vi "Rotate.vi"(2 "背景":dbl[][](array[numeric]), 3 "point":cluster{"x":i16, "y":i16} caption="位置", 4 "宽度":dbl, 5 "输入":cluster{"编号":i8, "方块":i32[][]}) -> (0 "输出":cluster{"编号":i8, "方块":i32[][]}, 1 "point 2":cluster{"x":i16, "y":i16} caption="新位置")   [LabVIEW 2010]
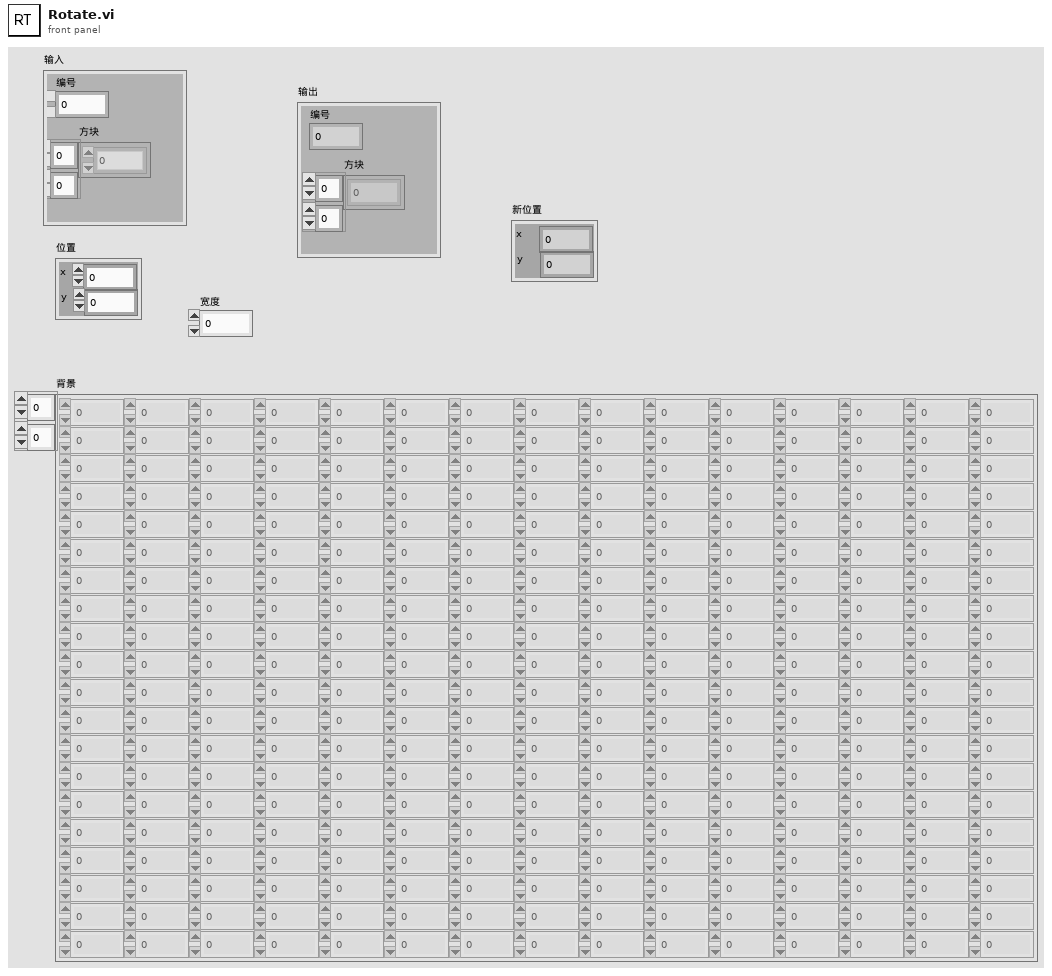
[diagram p1: front panel]
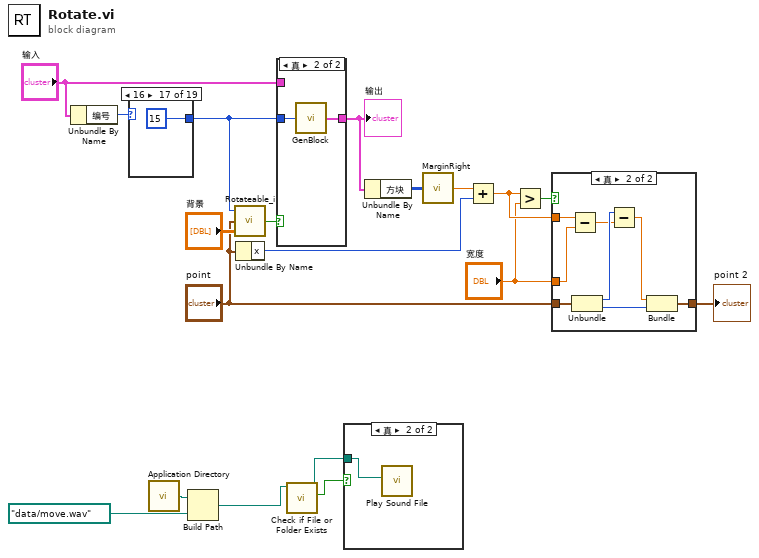
[diagram p0: block diagram]
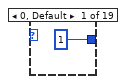
[diagram p5: hidden frame]
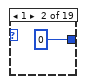
[diagram p6: hidden frame]
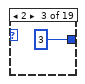
[diagram p7: hidden frame]
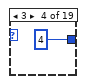
[diagram p8: hidden frame]
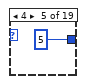
[diagram p9: hidden frame]
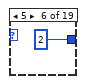
[diagram p10: hidden frame]
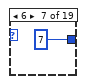
[diagram p11: hidden frame]
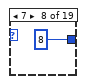
[diagram p12: hidden frame]
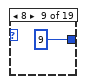
[diagram p13: hidden frame]
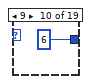
[diagram p14: hidden frame]
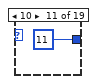
[diagram p15: hidden frame]
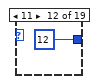
[diagram p16: hidden frame]
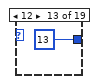
[diagram p17: hidden frame]
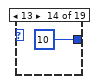
[diagram p18: hidden frame]
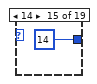
[diagram p19: hidden frame]
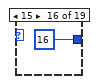
[diagram p20: hidden frame]
diagram:
  n1 = Unbundle By Name("输入") -> ("编号"=w16:i8)
  n2 = case shown="16" w16 {
    tunnel: [1 0 3 4 5 2 7 8 9 6 11 12 13 10 14 16 15 18 17] -> w15
    frame 0, Default {
    }
    frame 1 {
    }
    frame 2 {
    }
    frame 3 {
    }
    frame 4 {
    }
    frame 5 {
    }
    frame 6 {
    }
    frame 7 {
    }
    frame 8 {
    }
    frame 9 {
    }
    frame 10 {
    }
    frame 11 {
    }
    frame 12 {
    }
    frame 13 {
    }
    frame 14 {
    }
    frame 15 {
    }
    frame 16 {
    }
    frame 17 {
    }
    frame 18 {
    }
  }
  n3 = call <vilib>:"Application Directory.vi"() -> ("Application Directory"=w4:path)
  n4 = Build Path(base path=w4, name or relative path=path "data/move.wav") -> (appended path=w3:path)
  n5 = call "Rotateable_i.vi"("背景"="背景", "point"="point", "编号"=w15) -> ("Rotateable"=w18:bool)
  n6 = Unbundle By Name("point") -> ("x"=w12:i16)
  n7 = case shown="真" w18 {
    tunnel: [w39 w41] -> w11
    tunnel: "输入" -> [w39 _]
    tunnel: w15 -> [_ w40]
    frame False {
    }
    frame True {
      n8 = call "GenBlock.vi"("编号"=w40) -> ("输出"=w41:cluster{"编号":i8, "方块":i32[][]})
    }
  }
  "输出" <- w11
  n9 = call <vilib>:"Check if File or Folder Exists.vi"("path"=w3) -> ("file or folder exists?"=w2:bool, "dup path"=w1:path)  [unwired: 8 in, 1 out]
  n10 = case shown="真" w2 {
    tunnel: w1 -> [_ w42]
    frame False {
    }
    frame True {
      n11 = call <vilib>:"Play Sound File.vi"("path"=w42) -> ()  [unwired: 9 in, 2 out]
    }
  }
  n12 = Unbundle By Name(w11) -> ("方块"=w14:i32[][])
  n13 = call "MarginRight.vi"("输入"=w14) -> ("输出"=w13:dbl)
  n14 = Add(x=w13, y=w12) -> (x+y=w7:dbl)
  n15 = Greater?(x=w7, y="宽度") -> (0:w9:bool)
  n16 = case shown="真" w9 {
    tunnel: [w43 w50] -> w10
    tunnel: "point" -> [w43 w51]
    tunnel: w7 -> [_ w46]
    tunnel: "宽度" -> [_ w45]
    frame False {
    }
    frame True {
      n17 = Subtract(x=w46, y=w45) -> (x-y=w44:dbl)
      n18 = Unbundle(w51) -> ("x"=w48:i16, "y"=w49:i16)
      n19 = Subtract(x=w48, y=w44) -> (x-y=w47:dbl)
      n20 = Bundle(w47, "y"=w49) -> (w50:cluster{dbl, "y":i16})  [unwired: 1 in]
    }
  }
  "point 2" <- w10
